vi "NumatoRelay.Set Relay.vi"(8 "error in":errorcluster, 9 "State":bool, 10 "Relay":i32 min=0 max=7 step=1, 11 "VISA Alias":refnum<visa-resource-name>) -> (0 "error out":errorcluster, 3 "Write":string)   [LabVIEW 2018]
uses:
  <vilib>/Instr/_visa.llb/VISA Configure Serial Port (Instr).vi
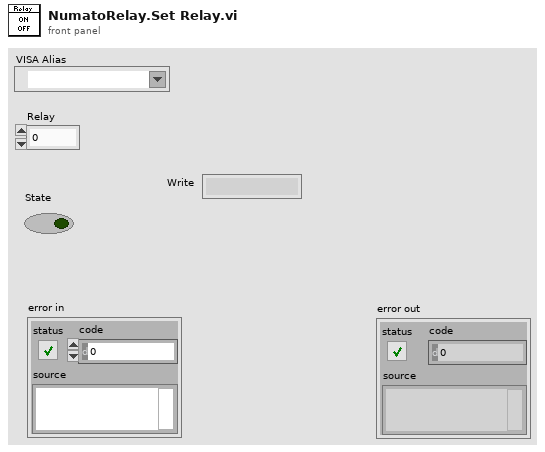
[diagram p1: front panel]
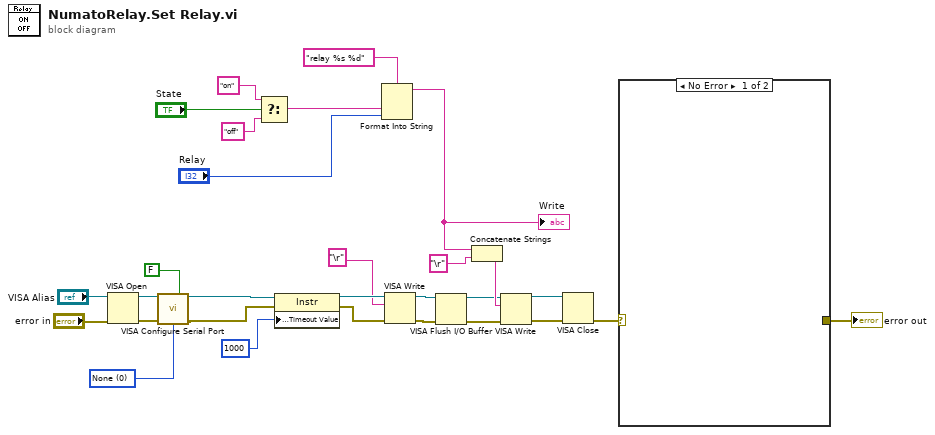
[diagram p0: block diagram]
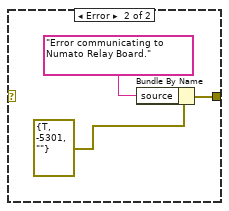
[diagram p2: hidden frame]
diagram:
  w16 = u16 0 items=["None", "XON/XOFF", "RTS/CTS", "XON/XOFF & RTS/CTS", "DTR/DSR", "XON/XOFF & DTR/DSR"] ("flow control (0:none)")
  n1 = VISA Open(error in (no error)="error in", VISA resource name="VISA Alias") -> (VISA resource name=w18:refnum<visa-resource-name>, error out=w17:errorcluster)  [unwired: 3 in]
  n2 = call-poly "VISA Configure Serial Port"("VISA resource name"=w18, "Enable Termination\nChar (T)"=FALSE ("Enable Termination\nChar (T)"), "error in (no error)"=w17, "flow control (0:none)"=w16) -> ("VISA resource name out"=w7:refnum<visa-resource-name>, "error out"=w6:errorcluster)  [unwired: 10 in]
  n3 = Select(t="on", s="State", f="off") -> (s? t:f=w19:string)
  n4 = property class="Instr"(reference=w7, error in=w6, "General Settings:Timeout Value"=u32 1000) -> (reference out=w13:refnum<visa-resource-name>, error out=w12:errorcluster)
  n5 = Format Into String(format string="relay %s %d", w19, "Relay") -> (resulting string=w15:string)  [unwired: 2 in, 1 out]
  "Write" <- w15
  n6 = VISA Write(VISA resource name=w13, write buffer="\r", error in (no error)=w12) -> (VISA resource name out=w11:refnum<visa-resource-name>, error out=w10:errorcluster)  [unwired: 1 out]
  n7 = VISA Flush I/O Buffer(VISA resource name=w11, error in (no error)=w10) -> (VISA resource name out=w8:refnum<visa-resource-name>, error out=w9:errorcluster)  [unwired: 1 in]
  n8 = Concatenate Strings(w15, "\r") -> (w14:string)
  n9 = VISA Write(VISA resource name=w8, write buffer=w14, error in (no error)=w9) -> (VISA resource name out=w1:refnum<visa-resource-name>, error out=w2:errorcluster)  [unwired: 1 out]
  n10 = VISA Close(VISA resource name=w1, error in (no error)=w2) -> (error out=w22:errorcluster)
  n11 = case shown="No Error" w22 {
    tunnel: [_ w30] -> w21
    frame No Error {
    }
    frame Error {
      n12 = Bundle By Name(cluster=errorcluster {"status"=TRUE, "code"=-5301, "source"=""} ("error constant"), "source"="Error communicating to Numato Relay Board.") -> (w30:errorcluster)
    }
  }
  "error out" <- w21
